vi "FGV tester data.vi"(10 "Enum(read)":enum16{"Write", "Read"}(ring)=enum."Read", 11 "data in":i16[](array[numeric])) -> (3 "data in 2":i16[](array[numeric]))   [LabVIEW 2018]
panel:
  in  "error in (no error)":errorcluster
  out "error out":errorcluster
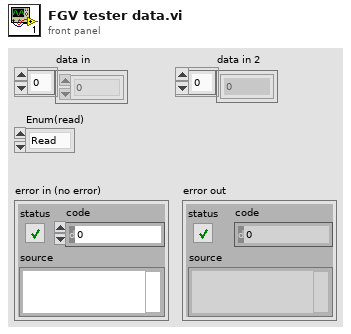
[diagram p1: front panel]
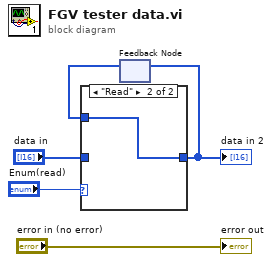
[diagram p0: block diagram]
diagram:
  n1 = feedback #1() -> (w4:i16[])  [unwired: 1 in]
  n2 = case shown="\"Read\"" "Enum(read)" {
    tunnel: [w6 w7] -> w2
    tunnel: w4 -> [_ w7]
    tunnel: "data in" -> [w6 _]
    frame "Write", Default {
    }
    frame "Read" {
    }
  }
  "data in 2" <- w2
  n3 = feedback-in #1(w2) -> ()
  "error out" <- "error in (no error)"
